vi "FEV_Strip & Build Path.vi"(7 "Strip Levels":i32, 8 "error in (no error)":errorcluster, 9 "Build Path":string, 11 "Path In":path) -> (0 "error out":errorcluster, 1 "Stripped Path":string, 3 "New Path Out":path)   [LabVIEW 2025]
doc: "Fetch VI/database path, especially for application and project."
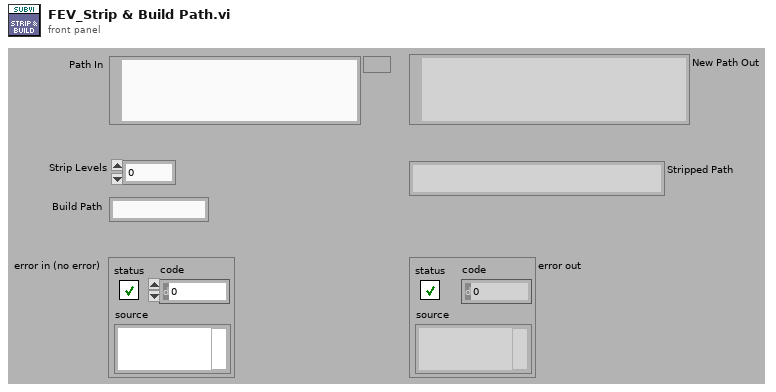
[diagram p1: front panel]
types:
  T1 = enum32{"invalid app kind", "Development System", "Run Time System", "Student Edition", "Embedded LabVIEW", "Evaluation", "Custom"}
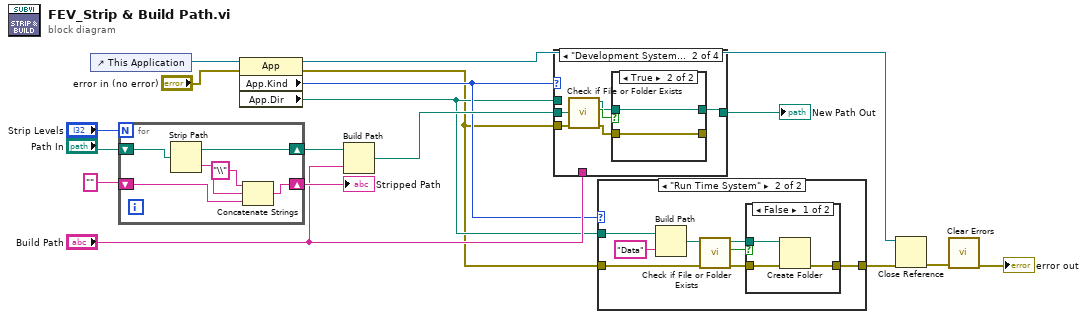
[diagram p0: block diagram]
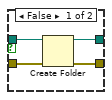
[diagram p5: hidden frame]
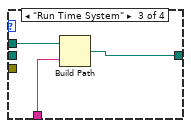
[diagram p6: hidden frame]
diagram:
  n1 = control-ref of="This Application"() -> (w6:refnum<vi>)
  n2 = for {
    N: "Strip Levels" -> [_]
    shift-right: [w22] -> w15
    shift-left: "Path In" -> [w23]
    shift-right: [w21] -> w14
    shift-left: "" -> [w20]
    n3 = Strip Path(path=w23) -> (stripped path=w22:path, name=w18:string)
    n4 = Concatenate Strings("\\" ("string"), w18, w20) -> (w21:string)
  }
  "Stripped Path" <- w14
  n5 = property class="App"(reference=w6, error in="error in (no error)") -> (reference out=w2:refnum<vi>, error out=w1:errorcluster, "App.Kind"=w9:T1, "App.Dir"=w8:path)
  n6 = Build Path(base path=w15, name or relative path="Build Path") -> (appended path=w12:path)
  n7 = case shown="\"Development System\"" w9 {
    tunnel: w12 -> [w24 w27 _ w40]
    tunnel: [w24 w25 w37 w40] -> w11
    tunnel: w8 -> [_ _ w39 _]
    tunnel: "Build Path" -> [_ _ w38 _]
    tunnel: w1 -> [_ w26 _ _]
    frame "invalid app kind", Default {
    }
    frame "Development System" {
      n8 = call <vilib>:"Check if File or Folder Exists.vi"("error in (no error)"=w26, "path"=w27) -> ("error out"=w28:errorcluster, "file or folder exists?"=w30:bool, "dup path"=w29:path)  [unwired: 7 in]
      n9 = case shown="True" w30 {
        tunnel: w29 -> [w34 w35]
        tunnel: w28 -> [w33 w36]
        tunnel: [w32 w36] -> _
        tunnel: [w31 w35] -> w25
        frame False {
          n10 = Create Folder(path (use dialog)=w34, error in=w33) -> (created path=w31:path, error out=w32:errorcluster)  [unwired: 1 in, 1 out]
        }
        frame True {
        }
      }
    }
    frame "Run Time System" {
      n11 = Build Path(base path=w39, name or relative path=w38) -> (appended path=w37:path)
    }
    frame "Evaluation" {
    }
  }
  "New Path Out" <- w11
  n12 = case shown="\"Run Time System\"" w9 {
    tunnel: w8 -> [_ w49]
    tunnel: w1 -> [w41 w46]
    tunnel: [w41 w42] -> w4
    frame "invalid app kind", Default {
    }
    frame "Run Time System" {
      n13 = Build Path(base path=w49, name or relative path="Data") -> (appended path=w47:path)
      n14 = call <vilib>:"Check if File or Folder Exists.vi"("error in (no error)"=w46, "path"=w47) -> ("error out"=w43:errorcluster, "file or folder exists?"=w45:bool, "dup path"=w44:path)  [unwired: 7 in]
      n15 = case shown="False" w45 {
        tunnel: w44 -> [w52 _]
        tunnel: w43 -> [w51 w53]
        tunnel: [w50 w53] -> w42
        frame False {
          n16 = Create Folder(path (use dialog)=w52, error in=w51) -> (error out=w50:errorcluster)  [unwired: 1 in, 2 out]
        }
        frame True {
        }
      }
    }
  }
  n17 = Close Reference(reference=w2, error in (no error)=w4) -> (error out=w3:errorcluster)
  n18 = call <vilib>:"Clear Errors.vi"("error in (no error)"=w3) -> ("error out"=→"error out":errorcluster)  [unwired: 5 in, 1 out]
